vi "MakeCross.vi"() -> ()   [LabVIEW 2014]
panel:
  in  "milliseconds to wait":u32
  in  "stop":bool
  in  "Amplitude (um)":dbl
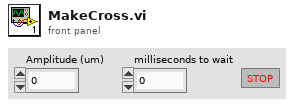
[diagram p1: front panel]
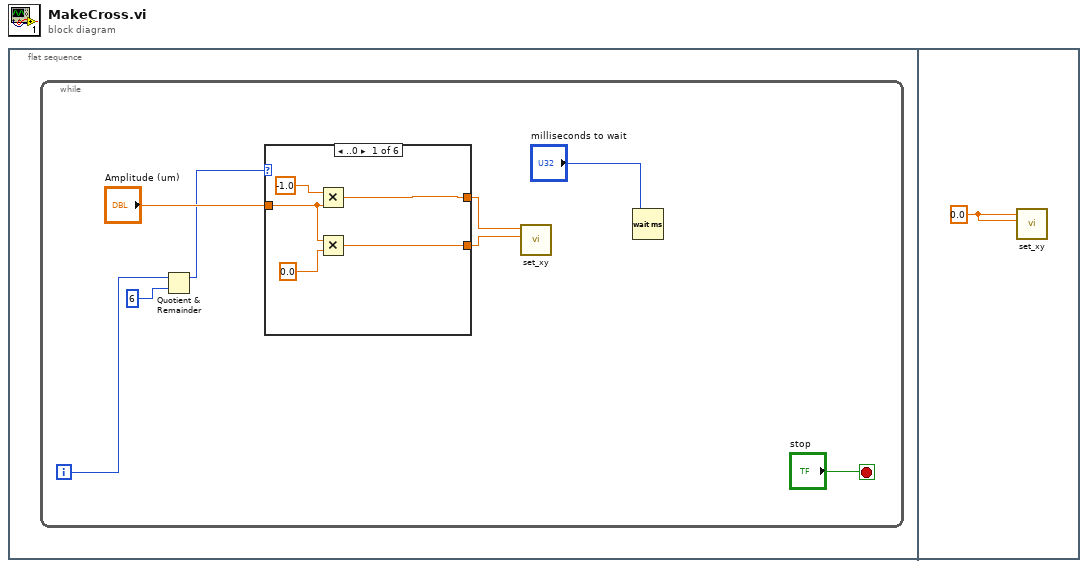
[diagram p0: block diagram]
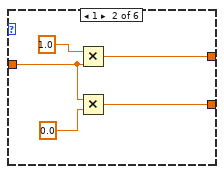
[diagram p2: hidden frame]
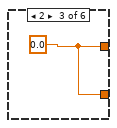
[diagram p3: hidden frame]
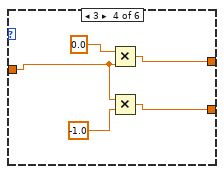
[diagram p4: hidden frame]
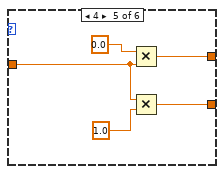
[diagram p5: hidden frame]
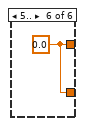
[diagram p6: hidden frame]
diagram:
  n1 = flat-sequence {
    frame #0 {
      n2 = while {
        i -> [w4]
        stop <- "stop" stop-if-true
        n3 = Quotient & Remainder(x=w4, y=6) -> (x-y*floor(x/y)=w2:i32)  [unwired: 1 out]
        n4 = case shown="..0" w2 {
          tunnel: "Amplitude (um)" -> [w11 w16 _ w22 w25 _]
          tunnel: [w10 w15 w19 w21 w27 w30] -> w6
          tunnel: [w9 w14 w19 w20 w26 w30] -> w5
          frame ..0 {
            n5 = Multiply(x=-1.0 ("y"), y=w11) -> (x*y=w10:dbl)
            n6 = Multiply(x=w11, y=0.0) -> (x*y=w9:dbl)
          }
          frame 1 {
            n7 = Multiply(x=1.0 ("y"), y=w16) -> (x*y=w15:dbl)
            n8 = Multiply(x=w16, y=0.0) -> (x*y=w14:dbl)
          }
          frame 2 {
            w19 = 0.0
          }
          frame 3 {
            n9 = Multiply(x=0.0 ("y"), y=w22) -> (x*y=w21:dbl)
            n10 = Multiply(x=w22, y=-1.0) -> (x*y=w20:dbl)
          }
          frame 4 {
            n11 = Multiply(x=0.0 ("y"), y=w25) -> (x*y=w27:dbl)
            n12 = Multiply(x=w25, y=1.0) -> (x*y=w26:dbl)
          }
          frame 5.. {
            w30 = 0.0
          }
        }
        n13 = call "set_xy.vi"("y_value_um"=w5, "x_value_um"=w6) -> ()  [unwired: 9 in, 1 out]
        n14 = Wait (ms)(milliseconds to wait="milliseconds to wait") -> ()  [unwired: 1 out]
      }
    }
    frame #1 {
      w31 = 0.0
      n15 = call "set_xy.vi"("y_value_um"=w31, "x_value_um"=w31) -> ()  [unwired: 9 in, 1 out]
    }
  }
